vi "startup.vi"(8 "error in (no error)":errorcluster, 11 "FringeTestingViewer in":refnum<class "FringeTestingViewer.lvclass">) -> (0 "error out":errorcluster, 3 "FringeTestingViewer out":refnum<class "FringeTestingViewer.lvclass">)   [LabVIEW 2009, in "Views.lvlib" / "Camera.lvlib" / "FringeTestingViewer.lvclass"]
uses:
  FringeTestingViewer.lvclass
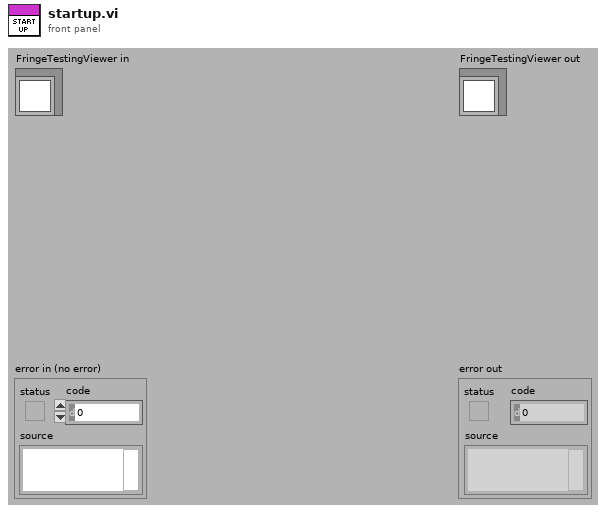
[diagram p1: front panel]
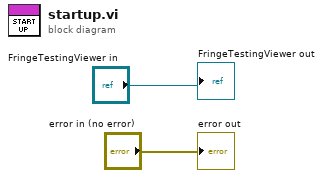
[diagram p0: block diagram]
diagram:
  "error out" <- "error in (no error)"
  "FringeTestingViewer out" <- "FringeTestingViewer in"
